vi "Directory to Tree.vi"(4 "Files found":i32(listbox)=1, 6 "error in":errorcluster, 7 "Level":i32=3, 8 "Path to start the search":path, 9 "Tree In":refnum<vi>) -> (0 "error out":errorcluster, 1 "Array of files found":path[](array[path]), 2 "Number of files found":i32, 3 "Tree Out":refnum<vi>)   [LabVIEW 2013, in "main.lvlib"]
doc: "This VI searches \"Path to start the search\" and all the path's subdirectories for files having names specified in \"Pattern to search\". This VI specifically does not search Windows shortcuts."
uses:
  main.lvlib
panel:
  in  "Parent Tag":string
  out "Working":bool=TRUE
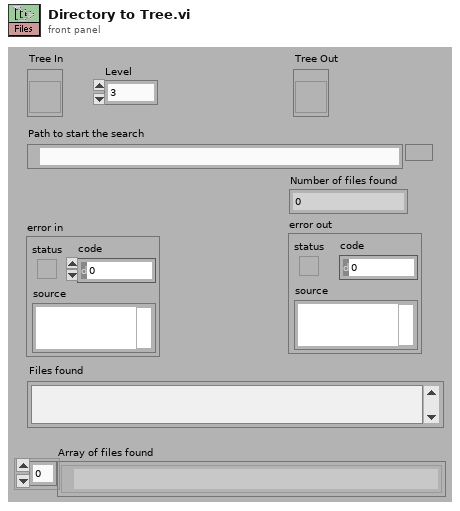
[diagram p1: front panel]
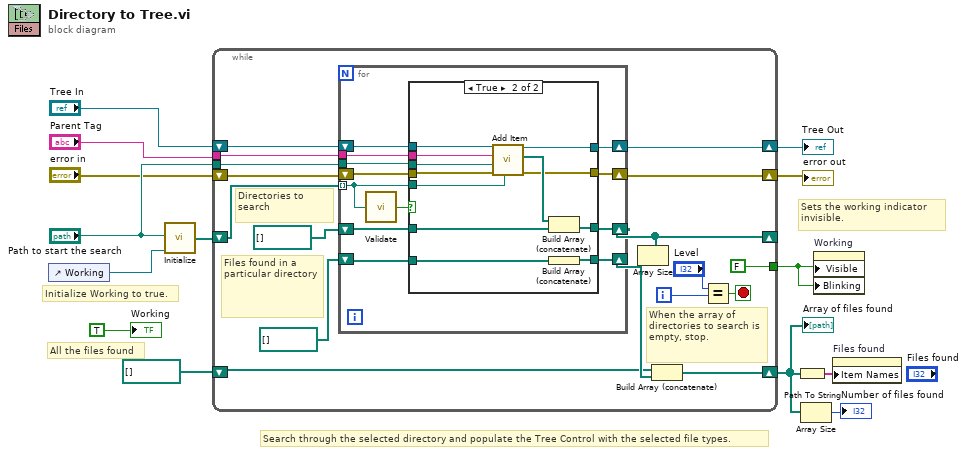
[diagram p0: block diagram]
diagram:
  # "Search through the selected directory and populate the Tree Control with the selected file types."
  # "Initialize Working to true."
  # "All the files found"
  # "Sets the working indicator invisible."
  n1 = control-ref of="Working"() -> (w6:refnum<vi>)
  n2 = call "Initialize.vi"("Working"=w6, "Path to start the search"="Path to start the search") -> ("Array"=w14:path[])  [unwired: 2 in]
  n3 = while {
    shift-right: [w30] -> _
    shift-left: w14 -> [w27]
    shift-right: [w31] -> w11
    shift-left: path[] [] -> [w25]
    tunnel: [FALSE] -> w8
    tunnel: "Parent Tag" -> [w22]
    tunnel: "Path to start the search" -> [w21]
    shift-right: [w18] -> w1
    shift-left: "error in" -> [w20]
    shift-right: [w19] -> w2
    shift-left: "Tree In" -> [w23]
    i -> [w15]
    stop <- w17 stop-if-true
    # "When the array of directories to search is empty, stop."
    # "Files found in a particular directory"
    # "Directories to search"
    n4 = for {
      tunnel: w27 -> [w39] mode=indexing
      shift-right: [w43] -> w30
      shift-left: path[] [] -> [w42]
      shift-right: [w40] -> w26
      shift-left: path[] [] -> [w41]
      tunnel: w22 -> [w36]
      tunnel: w21 -> [w35]
      shift-right: [w32] -> w18
      shift-left: w20 -> [w34]
      shift-right: [w33] -> w19
      shift-left: w23 -> [w37]
      n5 = call "Validate.vi"("Path"=w39) -> ("Valid Path?"=w38:bool)
      n6 = case shown="True" w38 {
        tunnel: [w47 w59] -> w43
        tunnel: w42 -> [w47 w58]
        tunnel: w41 -> [w46 w57]
        tunnel: [w46 w56] -> w40
        tunnel: w39 -> [_ w55]
        tunnel: w37 -> [w45 w51]
        tunnel: w36 -> [_ w49]
        tunnel: w35 -> [_ w48]
        tunnel: [w45 w50] -> w33
        tunnel: [w44 w52] -> w32
        tunnel: w34 -> [w44 w53]
        frame False {
          # "This file is either a shortcut or not a path"
        }
        frame True {
          n7 = call "Add Item.vi"("Path"=w55, "error in"=w53, "Path to start the search"=w48, "Parent Tag"=w49, "Tree In"=w51) -> ("error out"=w52:errorcluster, "Folders Found"=w54:path[], "Tree Out"=w50:refnum<vi>)  [unwired: 3 in]
          n8 = Build Array (concatenate)(w54, w58) -> (w59:path[])
          n9 = Build Array (concatenate)(w57) -> (w56:path[])
        }
      }
    }
    n10 = Array Size(array=w30) -> ()  [unwired: 1 out]
    n11 = Build Array (concatenate)(w25, w26) -> (w31:path[])
    n12 = Equal?(x="Level", y=w15) -> (x = y?=w17:bool)
  }
  "Array of files found" <- w11
  "error out" <- w1
  "Tree Out" <- w2
  n13 = Path To String(path=w11) -> (string=w13:string[])
  n14 = Array Size(array=w11) -> (size(s)=→"Number of files found":i32)
  n15 = property on="Working" class="Bool (strict)"("Visible"=w8, "Blinking"=w8) -> ()  [unwired: 2 in, 2 out]
  n16 = property on="Files found" class="LstBox (strict)"("Item Names"=w13) -> ()  [unwired: 2 in, 2 out]
  "Working" <- TRUE
